vi "SendFile.vi"(6 "Waveform Graph":waveform(i16)[](array[waveform])=[{"t0"=timestamp(0 s since 1904-01-01), "dt"=0.001, "Y"=[0, 17, 34, 50, 64, 77, 87, 94, 98, 100, 98, 94, 87, 77, 64, 50, 34, 17, 0, -17, -34, -50, -64, -77, -87, -94, -98, -100, -98, -94, -87, -77, -64, -50, -34, -17]}, {"t0"=timestamp(0 s since 1904-01-01), "dt"=0.001, "Y"=[100, 98, 94, 87, 77, 64, 50, 34, 17, 0, -17, -34, -50, -64, -77, -87, -94, -98, -100, -98, -94, -87, -77, -64, -50, -34, -17, 0, 17, 34, 50, 64, 77, 87, 94, 98]}]) -> (0 "error out":errorcluster)   [LabVIEW 2010]
panel:
  in  "meas_point":i32=4
  # "Добавилось или нет можно глянуть здесь\nhttp://smgr.alwaysdata.net/"
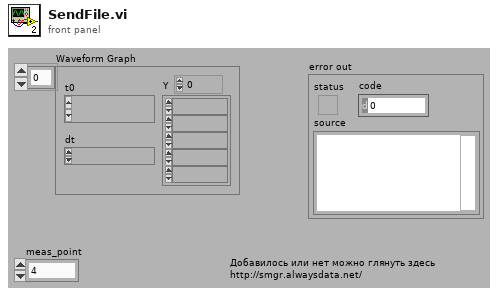
[diagram p1: front panel]
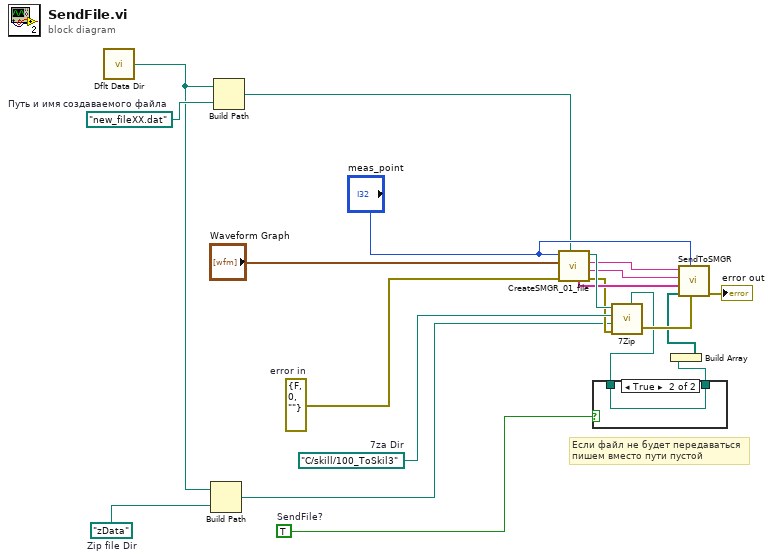
[diagram p0: block diagram]
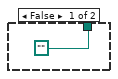
[diagram p2: hidden frame]
diagram:
  w9 = TRUE  # SendFile?
  w12 = errorcluster {"status"=FALSE, "code"=0, "source"=""}  # error in
  w5 = path "new_fileXX.dat"  # Путь и имя создаваемого файла
  w3 = path "zData"  # Zip file Dir
  w19 = path "C:/skill/100_ToSkil3"  # 7za Dir
  # "Если файл не будет передаваться\nпишем вместо пути пустой"
  n1 = call <vilib>:"Dflt Data Dir.vi"() -> ("App:Default Data Directory"=w4:path)
  n2 = Build Path(base path=w4, name or relative path=w3) -> (appended path=w2:path)
  n3 = Build Path(base path=w4, name or relative path=w5) -> (appended path=w6:path)
  n4 = call "CreateSMGR_01_file.vi"("file path to write"=w6, "error in"=w12, "Waveform Graph"="Waveform Graph", "meas_point"="meas_point") -> ("error out"=w14:errorcluster, "microseconds str"=w16:string, "date str"=w17:string, "file path out"=w20:path, "max_values"=w15:string[])  [unwired: 3 in]
  n5 = call "7Zip.vi"("error in"=w14, "Zip file Dir"=w2, "7za Dir"=w19, "File"=w20) -> ("error out"=w18:errorcluster, "new path"=w8:path)  [unwired: 1 in, 3 out]
  n6 = case shown="True" w9 {
    tunnel: w8 -> [_ w22]
    tunnel: [path "" w22] -> w7
    frame False {
    }
    frame True {
    }
  }
  n7 = Build Array(w7) -> (w1:path[])
  n8 = call "SendToSMGR.vi"("error in"=w18, "meas_point"="meas_point", "Files"=w1, "max_value_"=w15, "microseconds"=w16, "date"=w17) -> ("error out"=→"error out":errorcluster)  [unwired: 1 in, 4 out]
